vi "DHE_autoSample.vi"(5 "autoampling":bool=TRUE, 6 "error in":errorcluster, 7 "fd":i32, 10 "DHE_OBS":T1 {"exptime" format="%.2f"}, 11 "DBSRef":T2) -> (0 "post exposed frames":u16=1 min=1, 1 "pre-exposed frames":u16=1 min=1, 2 "mode":string, 4 "error out":errorcluster)   [LabVIEW 2016]
uses:
  DBSHAND/private/vis/DatabaseHand_RefNum.ctl
  DHE_Obs.ctl
  DBSHAND/private/vis/DatabaseHand_Element_Set(bool).vi
panel:
  in  "OutputType":string
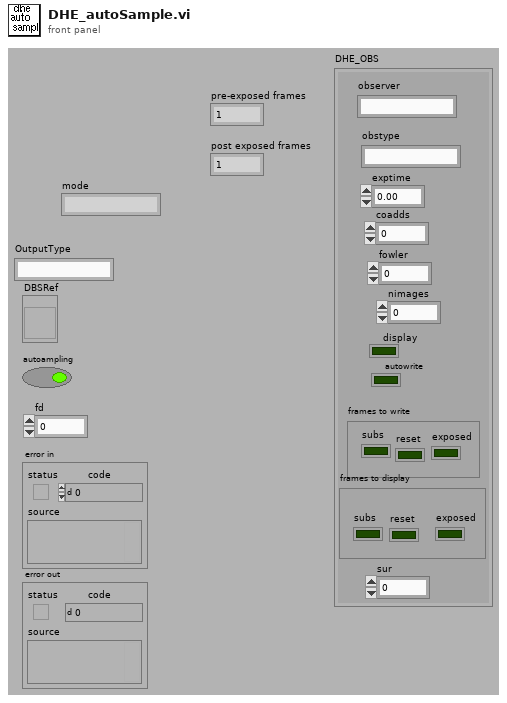
[diagram p1: front panel]
types:
  T1 = typedef "DHE_Obs.ctl" = cluster{"observer":string, "obstype":string, "exptime":dbl, "coadds":i32, "fowler":i32, "nimages":i32, "display":bool, "autowrite":bool, "frames to write":cluster{"subs":bool, "reset":bool, "exposed":bool}, "frames to display":cluster{"subs":bool, "reset":bool, "exposed":bool}, "sur":i32}
  T2 = typedef "DatabaseHand_RefNum.ctl" = refnum<vi>
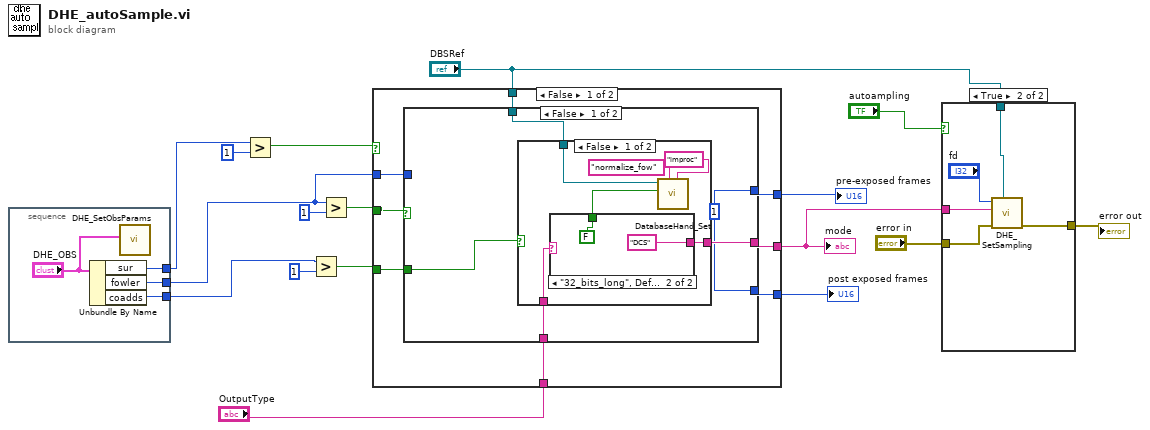
[diagram p0: block diagram]
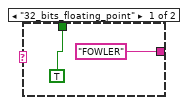
[diagram p3: hidden frame]
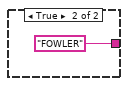
[diagram p4: hidden frame]
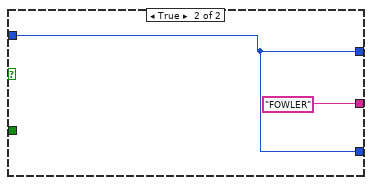
[diagram p5: hidden frame]
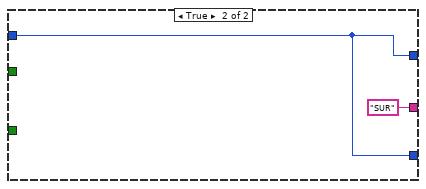
[diagram p6: hidden frame]
diagram:
  n1 = stacked-sequence {
    tunnel: [w21] -> w3
    tunnel: [w20] -> w2
    tunnel: [w19] -> w1
    frame #0 {
      n2 = Unbundle By Name("DHE_OBS") -> ("sur"=w21:i32, "fowler"=w20:i32, "coadds"=w19:i32)
      n3 = call "DHE_SetObsParams.vi"("DHE_OBS"="DHE_OBS") -> ()  [unwired: 11 out]
    }
  }
  n4 = Greater?(x=w3, y=u16 1) -> (0:w9:bool)
  n5 = Greater?(x=w1, y=u16 1) -> (0:w15:bool)
  n6 = Greater?(x=w2, y=u16 1) -> (0:w16:bool)
  n7 = case shown="False" w9 {
    tunnel: w16 -> [w29 _]
    tunnel: w15 -> [w28 _]
    tunnel: [w27 "SUR" ("t")] -> w6
    tunnel: [w26 w48] -> w13
    tunnel: w2 -> [w25 w48]
    tunnel: [w24 w48] -> w12
    tunnel: "OutputType" -> [w23 _]
    tunnel: "DBSRef" -> [w22 _]
    frame False {
      n8 = case shown="False" w29 {
        tunnel: [w34 "FOWLER" ("t")] -> w27
        tunnel: w28 -> [w33 _]
        tunnel: [w32 w46] -> w26
        tunnel: w25 -> [_ w46]
        tunnel: [w32 w46] -> w24
        tunnel: w23 -> [w31 _]
        tunnel: w22 -> [w30 _]
        frame False {
          w32 = 1
          n9 = case shown="False" w33 {
            tunnel: [w40 "FOWLER" ("t")] -> w34
            tunnel: w31 -> [w39 _]
            tunnel: w30 -> [w37 _]
            frame False {
              n10 = case shown="\"32_bits_long\", Default" w39 {
                tunnel: ["FOWLER" ("t") "DCS" ("t")] -> w40
                tunnel: [TRUE ("Normalize") FALSE ("Normalize")] -> w36
                frame "32_bits_floating_point" {
                }
                frame "32_bits_long", Default {
                }
              }
              n11 = call-poly "DatabaseHand_Set.vi"("group"="improc", "name"="normalize_fow" ("value"), "value"=w36, "Database RefNum in"=w37) -> ()  [unwired: 4 in, 4 out]
            }
            frame True {
            }
          }
        }
        frame True {
        }
      }
    }
    frame True {
    }
  }
  "mode" <- w6
  "post exposed frames" <- w12
  "pre-exposed frames" <- w13
  n12 = case shown="True" "autoampling" {
    tunnel: "DBSRef" -> [_ w55]
    tunnel: w6 -> [_ w53]
    tunnel: "error in" -> [w50 w52]
    tunnel: [w50 w51] -> w4
    frame False {
    }
    frame True {
      n13 = call "DHE_SetSampling.vi"("DBS Ref"=w55, "error in"=w52, "sampling type"=w53, "fd"="fd") -> ("error out"=w51:errorcluster)  [unwired: 7 out]
    }
  }
  "error out" <- w4
